vi "get Last Error.vi"() -> (3 "function return":string)   [LabVIEW 2012, in "cvlib.lvlib"]
doc: "extern \"C\" __declspec(dllexport) char* __cdecl getLastError();"
uses:
  cvlib.lvlib
  cvlib.dll
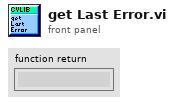
[diagram p1: front panel]
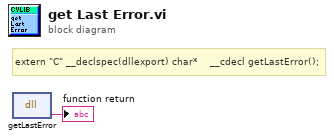
[diagram p0: block diagram]
diagram:
  # "extern \"C\" __declspec(dllexport) char* \t\t\t__cdecl getLastError();"
  n1 = dll-call lib="C:/Users/myerslab/workspace2/Libraries/ClearVolume/cpp/labview/lvcvlib/cvlib.*" fn="getLastError"() -> (→"function return":string)  [unwired: 3 in, 2 out]
